vi "PIDcontrol_y_axis.vi"() -> ()   [LabVIEW 2019]
uses:
  <vilib>/addons/control/pid/NI_PID_pid.lvlib
  <vilib>/addons/control/pid/pid.llb/PID Structure Conversion (DBL).vi
  <vilib>/addons/control/pid/pid.llb/PID (DBL).vi
panel:
  out "error out 4":errorcluster
  out "error out 3":errorcluster
  out "error out 2":errorcluster
  out "error out":errorcluster
  in  "Reinitialize":bool
  in  "stop":bool
  out "PID Out":dbl=1.8829840965238862 format="%0#4.1g"
  in  "PID Gains":T1={"Proportional Gain (Kc)"=0.8, "Integral Gain"=25.0, "Derivative Gain"=0.004}
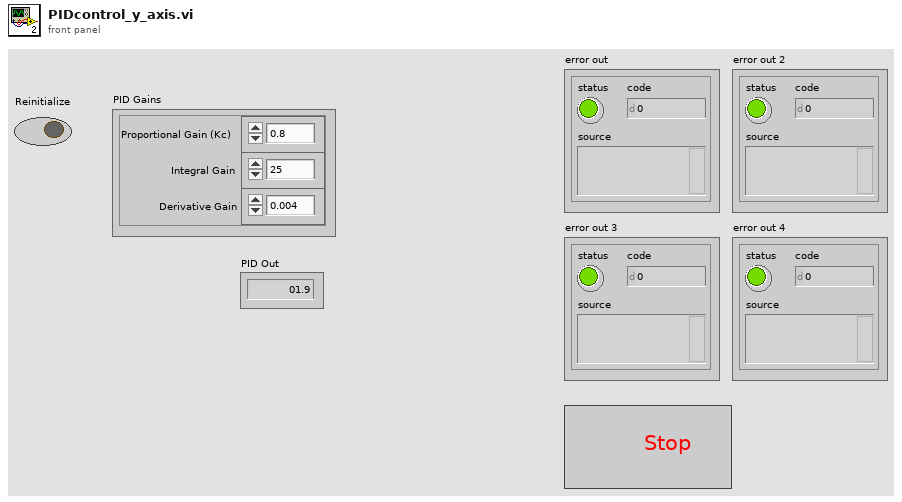
[diagram p1: front panel]
types:
  T1 = cluster{"Proportional Gain (Kc)":dbl, "Integral Gain":dbl, "Derivative Gain":dbl}
  T2 = enum16{"Academic (Standard)", "Parallel", "Series"}
  T3 = cluster{"proportional gain (Kc)":dbl, "integral time (Ti, min)":dbl, "derivative time (Td, min)":dbl}
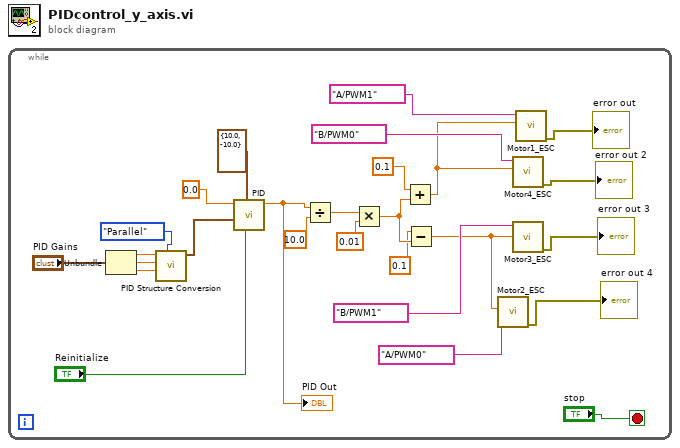
[diagram p0: block diagram]
diagram:
  n1 = while {
    stop <- "stop" stop-if-true
    n2 = Unbundle("PID Gains") -> ("Proportional Gain (Kc)"=w24:dbl, "Integral Gain"=w25:dbl, "Derivative Gain"=w26:dbl)
    n3 = call-poly <vilib>:"PID Structure Conversion.vi"("PID structure"=T2."Parallel", "derivative"=w26, "integral"=w25, "proportional"=w24) -> ("PID gains"=w20:T3)  [unwired: 7 in]
    n4 = call-poly <vilib>:"PID.vi"("reinitialize? (F)"="Reinitialize", "output range"=cluster{"output high":dbl, "output low":dbl} {"output high"=10.0, "output low"=-10.0}, "PID gains"=w20, "setpoint"=0.0 ("Angle (rads)")) -> ("output"=w18:dbl)  [unwired: 6 in, 1 out]
    "PID Out" <- w18
    n5 = Divide(x=w18, y=10.0) -> (x/y=w17:dbl)
    n6 = Multiply(x=w17, y=0.01) -> (x*y=w16:dbl)
    n7 = Add(x=0.1, y=w16) -> (x+y=w1:dbl)
    n8 = Subtract(x=0.1, y=w16) -> (x-y=w2:dbl)
    n9 = call "Motor2_ESC.vi"("Percent Power"=w2, "Channel Name"=tag "A/PWM0") -> ("error out"=→"error out 4":errorcluster)  [unwired: 9 in]
    n10 = call "Motor4_ESC.vi"("Percent Power"=w1, "Channel Name"=tag "B/PWM0") -> ("error out"=→"error out 2":errorcluster)  [unwired: 9 in]
    n11 = call "Motor3_ESC.vi"("Percent Power"=w2, "Channel Name"=tag "B/PWM1") -> ("error out"=→"error out 3":errorcluster)  [unwired: 9 in]
    n12 = call "Motor1_ESC.vi"("Percent Power"=w1, "Channel Name"=tag "A/PWM1") -> ("error out"=→"error out":errorcluster)  [unwired: 9 in]
  }
